vi "CTR_to_DutyCycle.vi"(2 "LOW CTR":u32, 3 "HIGH CTR":u32) -> (0 "duty cycle [%]":dbl, 1 "period [s]":dbl)   [LabVIEW 2016]
panel:
  in  "Ticks per second (40 MHz)":dbl=25000000.0 format="%#_13g"
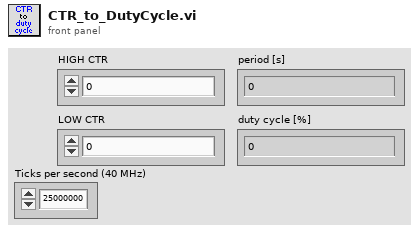
[diagram p1: front panel]
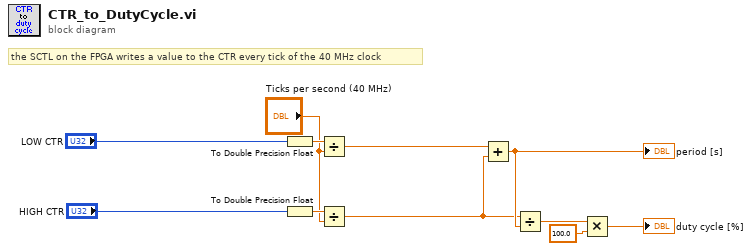
[diagram p0: block diagram]
diagram:
  # "the SCTL on the FPGA writes a value to the CTR every tick of the 40 MHz clock"
  n1 = To Double Precision Float(number="LOW CTR") -> (double precision float=w6:dbl)
  n2 = To Double Precision Float(number="HIGH CTR") -> (double precision float=w7:dbl)
  n3 = Divide(x=w6, y="Ticks per second (40 MHz)") -> (x/y=w4:dbl)
  n4 = Divide(x=w7, y="Ticks per second (40 MHz)") -> (x/y=w3:dbl)
  n5 = Add(x=w4, y=w3) -> (x+y=w9:dbl)
  "period [s]" <- w9
  n6 = Divide(x=w3, y=w9) -> (x/y=w2:dbl)
  n7 = Multiply(x=w2, y=100.0) -> (x*y=→"duty cycle [%]":dbl)
